vi "Teleop.vi"(10 "Match Info":T1={"Autonomous Elapsed Seconds"=0.0, "TeleOp Elapsed Seconds"=0.0, "Disabled Elapsed Seconds"=0.0, "Visited Autonomous"=FALSE, "Visited TeleOp"=FALSE, "Visited Disabled"=FALSE, "Autonomous Settings"={"Autonomous Style"=enum."Independent", "VI Refnum"=refnum}}, 11 "Call Context":T2) -> ()   [LabVIEW 2012]
doc: "This VI is called for each TeleOp packet received from the DS where the robot is not disabled. It is often used to read from the joysticks and update I/O or to update setpoints for timed control loops. It should complete and return within 20 milliseconds or it may miss DS packets."
uses:
  <vilib>/Rock Robotics/WPI/DriverStation/WPI_DriverStationDerivedRobotMode.ctl
  <vilib>/Rock Robotics/WPI/DriverStation/WPI_DriverStationMatch Info.ctl
  Robot Global Data.vi
  <vilib>/Rock Robotics/WPI/Joystick/WPI_JoystickGetSetRefNum.vi
  <vilib>/Rock Robotics/WPI/RobotDrive/WPI_RobotDriveGetSetRefNum.vi
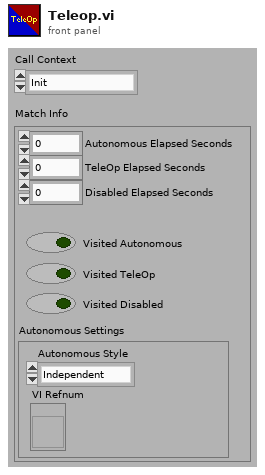
[diagram p1: front panel]
types:
  T1 = typedef "WPI_DriverStationMatch Info.ctl" = cluster{"Autonomous Elapsed Seconds":dbl, "TeleOp Elapsed Seconds":dbl, "Disabled Elapsed Seconds":dbl, "Visited Autonomous":bool, "Visited TeleOp":bool, "Visited Disabled":bool, "Autonomous Settings":cluster{"Autonomous Style":enum16{"Iterative", "Independent"}, "VI Refnum":refnum<vi>}}
  T2 = typedef "WPI_DriverStationDerivedRobotMode.ctl" = enum16{"Init", "Execute", "Stop"}
  T3 = typedef "WPI_RobotDriveDevRef.ctl" = cluster{"DevStatus":errorcluster, "Motors[]":T4[], "Square Inputs":bool, "Max Output":dbl, "Isochronous":bool}
  T4 = typedef "WPI_MotorControlDeviceRef.ctl" = cluster{"DeviceStatus":errorcluster, "Type":enum16{"PWM", "CAN"}, "PWM":cluster{"Digital Module":T5, "PWM Channel":T6, "DeadBand":T7}, "CAN":cluster{"Device Number":u8, "Control Mode":T8, "Semaphore":T9, "Max Vout":dbl}, "Invert":bool, "TransformRef":T10, "InvTransformRef":T10}
  T5 = typedef "FPGA_TypedefDigitalModule.ctl" = enum16{"Digital Module 1", "Digital Module 2"}
  T6 = typedef "FPGA_DIOPWMChannel.ctl" = enum8{"PWM 1", "PWM 2", "PWM 3", "PWM 4", "PWM 5", "PWM 6", "PWM 7", "PWM 8", "PWM 9", "PWM 10", "Invalid"}
  T7 = typedef "WPI_PWMDeadband.ctl" = cluster{"Name":string, "maxPositivePwm":i32, "minPositivePwm":i32, "centerPwm":i32, "maxNegativePwm":i32, "minNegativePwm":i32, "angularRange":u16}
  T8 = typedef "WPI_CANJaguar_ControlMode.ctl" = enum8{"Percent VBus", "Current", "Speed", "Position", "Voltage"}
  T9 = typedef "Semaphore RefNum" = refnum<k1>
  T10 = typedef "WPI_PWMTransform_ConPane.ctl" = refnum<vi>
  T11 = typedef "WPI_JoystickDevRef.ctl" = cluster{"Device":T12}
  T12 = typedef "WPI_JoystickDeviceEnum.ctl" = enum16{"USB 1", "USB 2", "USB 3", "USB 4", "Kinect 1", "Kinect 2"}
  T13 = typedef "WPI_JoystickButtonState.ctl" = cluster{"Button 1":bool, "Button 2":bool, "Button 3":bool, "Button 4":bool, "Button 5":bool, "Button 6":bool, "Button 7":bool, "Button 8":bool, "Button 9":bool, "Button 10":bool, "Button 11":bool, "Button 12":bool}
  T14 = cluster{"axis 1 (x)":dbl, "axis 2 (y)":dbl, "axis 3 (throttle)":dbl, "axis 4":dbl, "axis 5":dbl, "axis 6":dbl}
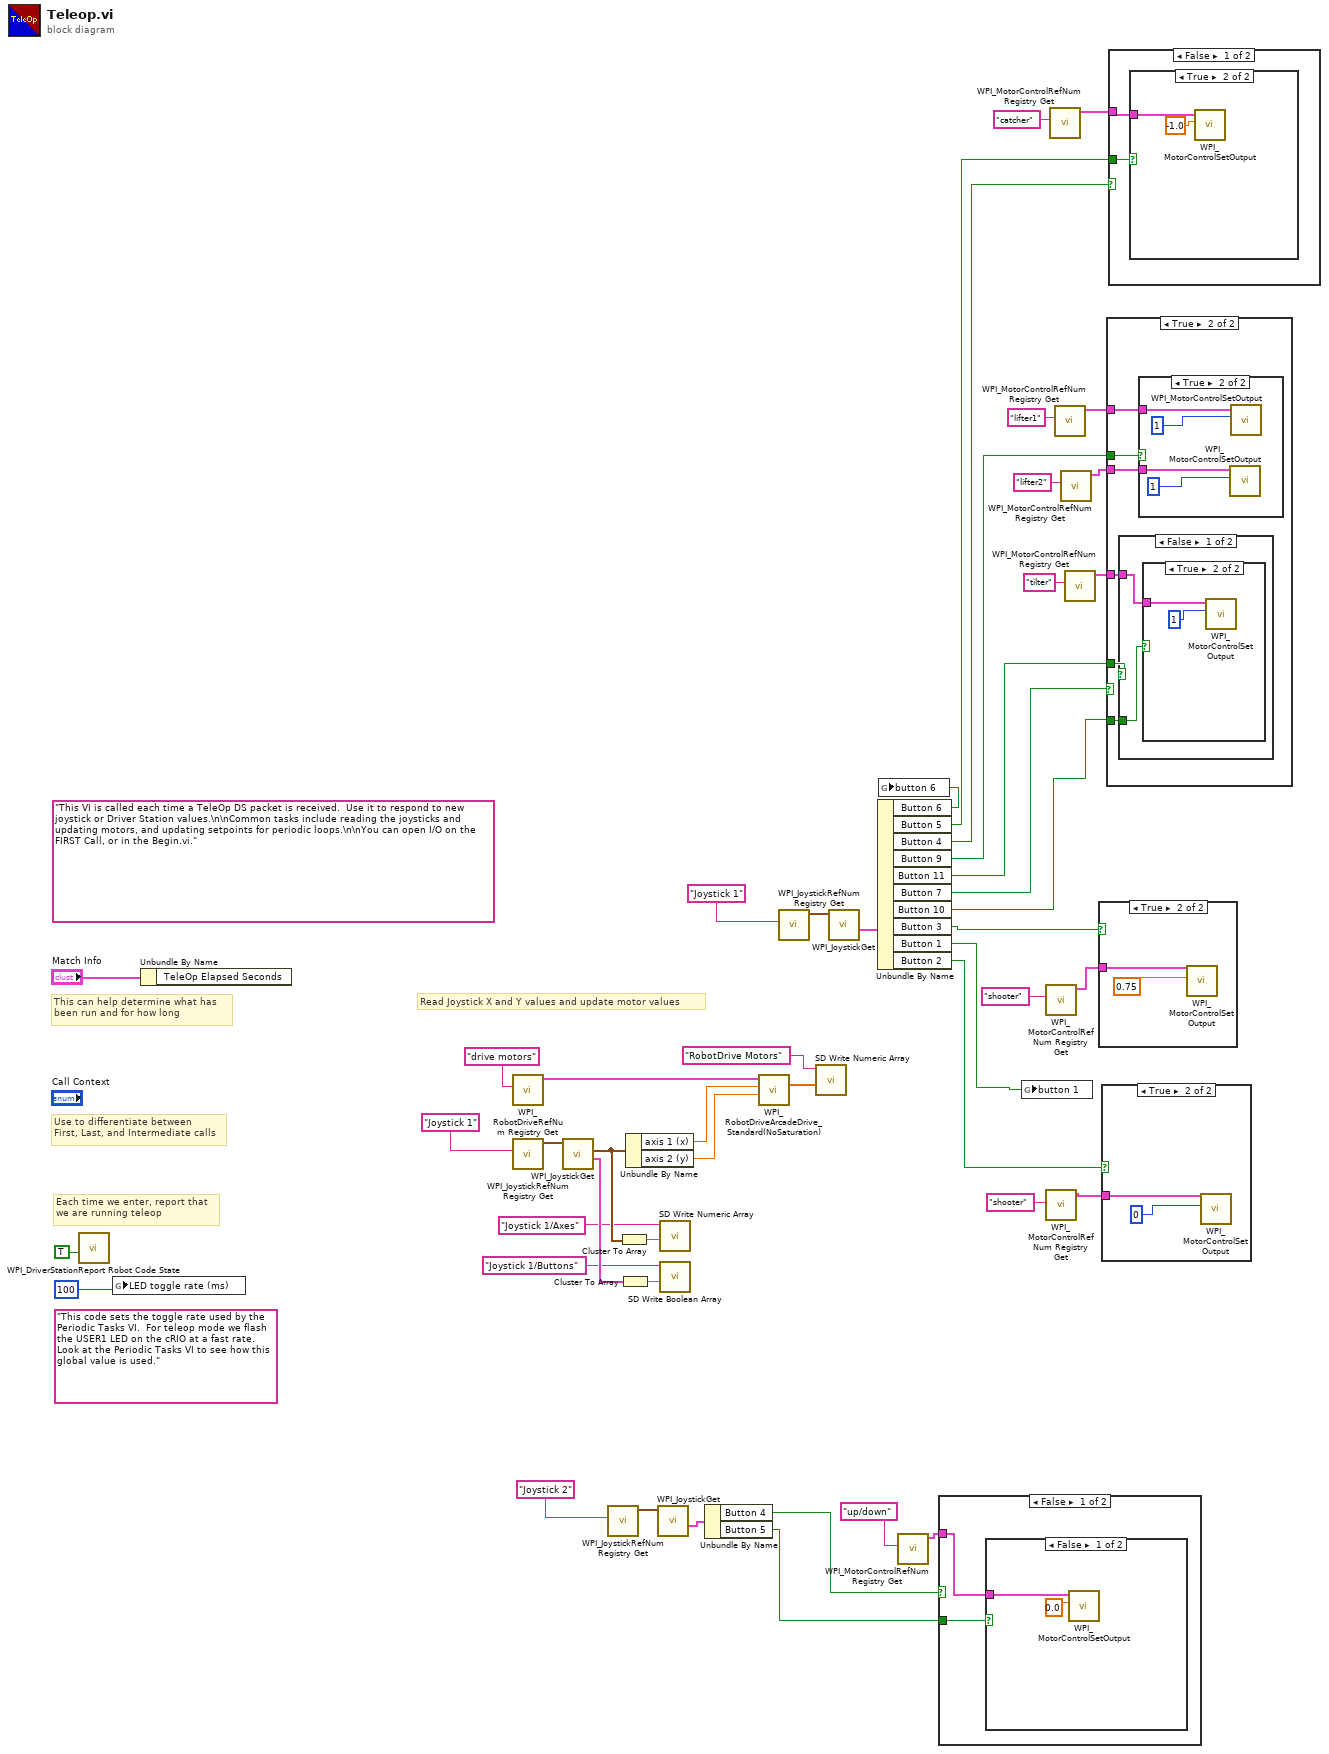
[diagram p0: block diagram]
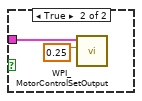
[diagram p2: hidden frame]
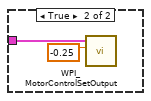
[diagram p3: hidden frame]
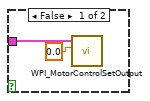
[diagram p4: hidden frame]
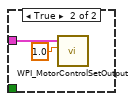
[diagram p5: hidden frame]
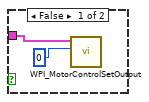
[diagram p7: hidden frame]
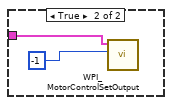
[diagram p8: hidden frame]
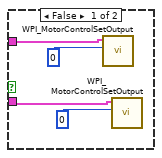
[diagram p9: hidden frame]
diagram:
  (unwired) "This code sets the toggle rate used by the Periodic Tasks VI.  For teleop mode we flash the USER1 LED on the cRIO at a fast rate.  Look at the Periodic Tasks VI to see how this global value is used."
  (unwired) "This VI is called each time a TeleOp DS packet is received.  Use it to respond to new joystick or Driver Station values.\n\nCommon tasks include reading the joysticks and updating motors, and updating setpoints for periodic loops.\n\nYou can open I/O on the FIRST Call, or in the Begin.vi."
  # "Each time we enter, report that\nwe are running teleop"
  # "Use to differentiate between\nFirst, Last, and Intermediate calls"
  # "This can help determine what has\nbeen run and for how long"
  # "Read Joystick X and Y values and update motor values"
  n1 = call <vilib>:"WPI_DriverStationReport Robot Code State.vi"("TeleOp"=TRUE ("Autonomous")) -> ()  [unwired: 10 in, 1 out]
  n2 = global write "Robot Global Data.vi" "LED toggle rate (ms)"(u32 100 ("LED ms toggle rate")) -> ()
  n3 = Unbundle By Name("Match Info") -> ()  [unwired: 1 out]
  n4 = call <vilib>:"WPI_RobotDriveRefNum Registry Get.vi"("refnum name"="drive motors") -> ("RobotDriveDevRef"=w47:T3)  [unwired: 1 in, 9 out]
  n5 = call <vilib>:"WPI_JoystickRefNum Registry Get.vi"("refnum name"="Joystick 1") -> ("JoystickDevRef"=w43:T11)  [unwired: 1 in, 9 out]
  n6 = call <vilib>:"WPI_JoystickGet.vi"("JoystickDevRef"=w43) -> ("Buttons"=w40:T13, "Axes"=w37:T14)  [unwired: 1 in, 4 out]
  n7 = call <vilib>:"WPI_JoystickRefNum Registry Get.vi"("refnum name"="Joystick 2") -> ("JoystickDevRef"=w6:T11)  [unwired: 1 in, 9 out]
  n8 = Cluster To Array(cluster=w37) -> (array=w36:dbl[])
  n9 = Cluster To Array(cluster=w40) -> (array=w39:bool[])
  n10 = Unbundle By Name(w37) -> ("axis 1 (x)"=w46:dbl, "axis 2 (y)"=w45:dbl)
  n11 = call <vilib>:"WPI_JoystickGet.vi"("JoystickDevRef"=w6) -> ("Buttons"=w5:T13)  [unwired: 1 in, 5 out]
  n12 = call <vilib>:"SD Write Numeric Array.vi"("Numeric Array"=w36, "Name"="Joystick 1/Axes") -> ()  [unwired: 8 in, 2 out]
  n13 = call <vilib>:"SD Write Boolean Array.vi"("Boolean Array"=w39, "Name"="Joystick 1/Buttons") -> ()  [unwired: 8 in, 2 out]
  n14 = Unbundle By Name(w5) -> ("Button 4"=w4:bool, "Button 5"=w1:bool)
  n15 = call <vilib>:"WPI_RobotDriveArcadeDrive_Standard(NoSaturation).vi"("Y axis value"=w45, "X axis value"=w46, "RobotDriveDevRef"=w47) -> ("Motor Values"=w33:dbl[])  [unwired: 1 in, 7 out]
  n16 = call <vilib>:"WPI_JoystickRefNum Registry Get.vi"("refnum name"="Joystick 1") -> ("JoystickDevRef"=w31:T11)  [unwired: 1 in, 9 out]
  n17 = call <vilib>:"SD Write Numeric Array.vi"("Numeric Array"=w33, "Name"="RobotDrive Motors") -> ()  [unwired: 8 in, 2 out]
  n18 = call <vilib>:"WPI_JoystickGet.vi"("JoystickDevRef"=w31) -> ("Buttons"=w30:T13)  [unwired: 1 in, 5 out]
  n19 = Unbundle By Name(w30) -> ("Button 6"=w14:bool, "Button 5"=w13:bool, "Button 4"=w12:bool, "Button 9"=w18:bool, "Button 11"=w23:bool, "Button 7"=w16:bool, "Button 10"=w17:bool, "Button 3"=w29:bool, "Button 1"=w15:bool, "Button 2"=w26:bool)
  n20 = global write "Robot Global Data.vi" "button 6"(w14) -> ()
  n21 = call <vilib>:"WPI_MotorControlRefNum Registry Get.vi"("refnum name"="up/down") -> ("MotorControlDevRef"=w2:T4)  [unwired: 9 in, 1 out]
  n22 = case shown="False" w4 {
    tunnel: w2 -> [w51 w57]
    tunnel: w1 -> [w50 _]
    frame False {
      n23 = case shown="False" w50 {
        tunnel: w51 -> [w52 w54]
        frame False {
          n24 = call <vilib>:"WPI_MotorControlSetOutput.vi"("Output"=0.0, "MotorControlDevRef"=w52) -> ()  [unwired: 7 in, 3 out]
        }
        frame True {
          n25 = call <vilib>:"WPI_MotorControlSetOutput.vi"("Output"=0.25, "MotorControlDevRef"=w54) -> ()  [unwired: 7 in, 3 out]
        }
      }
    }
    frame True {
      n26 = call <vilib>:"WPI_MotorControlSetOutput.vi"("Output"=-0.25, "MotorControlDevRef"=w57) -> ()  [unwired: 7 in, 3 out]
    }
  }
  n27 = global write "Robot Global Data.vi" "button 1"(w15) -> ()
  n28 = call <vilib>:"WPI_MotorControlRefNum Registry Get.vi"("refnum name"="shooter") -> ("MotorControlDevRef"=w27:T4)  [unwired: 9 in, 1 out]
  n29 = call <vilib>:"WPI_MotorControlRefNum Registry Get.vi"("refnum name"="shooter") -> ("MotorControlDevRef"=w25:T4)  [unwired: 9 in, 1 out]
  n30 = call <vilib>:"WPI_MotorControlRefNum Registry Get.vi"("refnum name"="catcher") -> ("MotorControlDevRef"=w10:T4)  [unwired: 9 in, 1 out]
  n31 = call <vilib>:"WPI_MotorControlRefNum Registry Get.vi"("refnum name"="lifter1") -> ("MotorControlDevRef"=w20:T4)  [unwired: 9 in, 1 out]
  n32 = call <vilib>:"WPI_MotorControlRefNum Registry Get.vi"("refnum name"="lifter2") -> ("MotorControlDevRef"=w19:T4)  [unwired: 9 in, 1 out]
  n33 = call <vilib>:"WPI_MotorControlRefNum Registry Get.vi"("refnum name"="tilter") -> ("MotorControlDevRef"=w8:T4)  [unwired: 9 in, 1 out]
  n34 = case shown="True" w29 {
    tunnel: w27 -> [_ w59]
    frame False {
    }
    frame True {
      n35 = call <vilib>:"WPI_MotorControlSetOutput.vi"("Output"=0.75, "MotorControlDevRef"=w59) -> ()  [unwired: 7 in, 3 out]
    }
  }
  n36 = case shown="True" w26 {
    tunnel: w25 -> [_ w60]
    frame False {
    }
    frame True {
      n37 = call <vilib>:"WPI_MotorControlSetOutput.vi"("Output"=0, "MotorControlDevRef"=w60) -> ()  [unwired: 7 in, 3 out]
    }
  }
  n38 = case shown="True" w16 {
    tunnel: w17 -> [_ w63]
    tunnel: w23 -> [_ w64]
    tunnel: w20 -> [_ w67]
    tunnel: w19 -> [_ w66]
    tunnel: w18 -> [_ w65]
    tunnel: w8 -> [_ w62]
    frame False {
    }
    frame True {
      n39 = case shown="False" w64 {
        tunnel: w63 -> [w69 _]
        tunnel: w62 -> [w68 w74]
        frame False {
          n40 = case shown="True" w69 {
            tunnel: w68 -> [w70 w72]
            frame False {
              n41 = call <vilib>:"WPI_MotorControlSetOutput.vi"("Output"=0, "MotorControlDevRef"=w70) -> ()  [unwired: 7 in, 3 out]
            }
            frame True {
              n42 = call <vilib>:"WPI_MotorControlSetOutput.vi"("Output"=1, "MotorControlDevRef"=w72) -> ()  [unwired: 7 in, 3 out]
            }
          }
        }
        frame True {
          n43 = call <vilib>:"WPI_MotorControlSetOutput.vi"("Output"=-1, "MotorControlDevRef"=w74) -> ()  [unwired: 7 in, 3 out]
        }
      }
      n44 = case shown="True" w65 {
        tunnel: w67 -> [w78 w81]
        tunnel: w66 -> [w76 w80]
        frame False {
          n45 = call <vilib>:"WPI_MotorControlSetOutput.vi"("Output"=0, "MotorControlDevRef"=w78) -> ()  [unwired: 7 in, 3 out]
          n46 = call <vilib>:"WPI_MotorControlSetOutput.vi"("Output"=0, "MotorControlDevRef"=w76) -> ()  [unwired: 7 in, 3 out]
        }
        frame True {
          n47 = call <vilib>:"WPI_MotorControlSetOutput.vi"("Output"=1, "MotorControlDevRef"=w80) -> ()  [unwired: 7 in, 3 out]
          n48 = call <vilib>:"WPI_MotorControlSetOutput.vi"("Output"=1, "MotorControlDevRef"=w81) -> ()  [unwired: 7 in, 3 out]
        }
      }
    }
  }
  n49 = case shown="False" w12 {
    tunnel: w13 -> [w85 _]
    tunnel: w10 -> [w84 w91]
    frame False {
      n50 = case shown="True" w85 {
        tunnel: w84 -> [w86 w88]
        frame False {
          n51 = call <vilib>:"WPI_MotorControlSetOutput.vi"("Output"=0.0, "MotorControlDevRef"=w86) -> ()  [unwired: 7 in, 3 out]
        }
        frame True {
          n52 = call <vilib>:"WPI_MotorControlSetOutput.vi"("Output"=-1.0, "MotorControlDevRef"=w88) -> ()  [unwired: 7 in, 3 out]
        }
      }
    }
    frame True {
      n53 = call <vilib>:"WPI_MotorControlSetOutput.vi"("Output"=1.0, "MotorControlDevRef"=w91) -> ()  [unwired: 7 in, 3 out]
    }
  }
